vi "发送.vi"(8 "error in (no error)":errorcluster caption="错误输入（无错误）", 10 "消息类.lvclass":refnum<class "消息类.lvclass">, 11 "VISA 输入":refnum<class "VISA.lvclass">) -> (0 "error out":errorcluster caption="错误输出", 3 "VISA 输出":refnum<class "VISA.lvclass">)   [LabVIEW 2016, in "VISA.lvclass"]
uses:
  VISA.lvclass
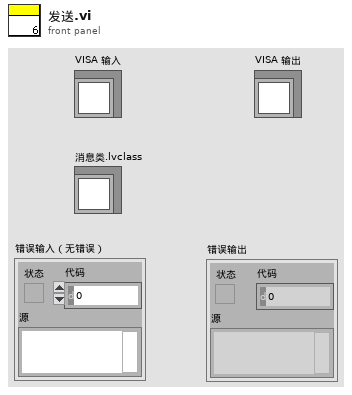
[diagram p1: front panel]
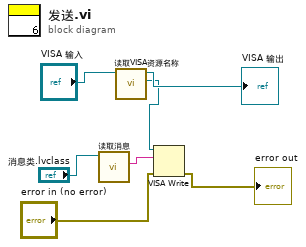
[diagram p0: block diagram]
diagram:
  n1 = call-dynamic "读取消息.vi"("消息类输入"="消息类.lvclass") -> ("消息"=w4:string)  [unwired: 8 in, 2 out]
  n2 = call-dynamic "读取VISA资源名称.vi"("VISA输入"="VISA 输入") -> ("VISA资源名称"=w5:refnum<visa-resource-name>, "VISA输出"=→"VISA 输出":refnum<class "VISA.lvclass">)  [unwired: 8 in, 1 out]
  n3 = VISA Write(VISA resource name=w5, write buffer=w4, error in (no error)="error in (no error)") -> (error out=→"error out":errorcluster)  [unwired: 2 out]
